vi "hipotTest.vi"() -> ()   [LabVIEW 2022 SP3]
uses:
  <vilib>/regexp/Match Regular Expression.xnode
panel:
  in  "?":bool
  out "HIPOT":bool
  out "HIPOT_R":string="FAIL"
  out "HIPOT BUFFER":string
  in  "start_hipot":bool
  in  "error in (no error)":errorcluster
  in  "VISA_TEST_L":refnum<visa-resource-name>="COM2"
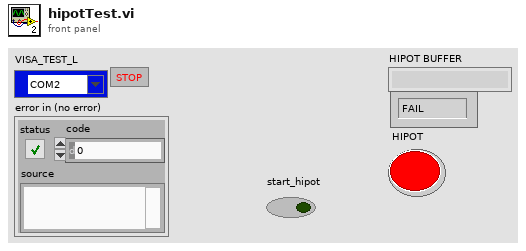
[diagram p1: front panel]
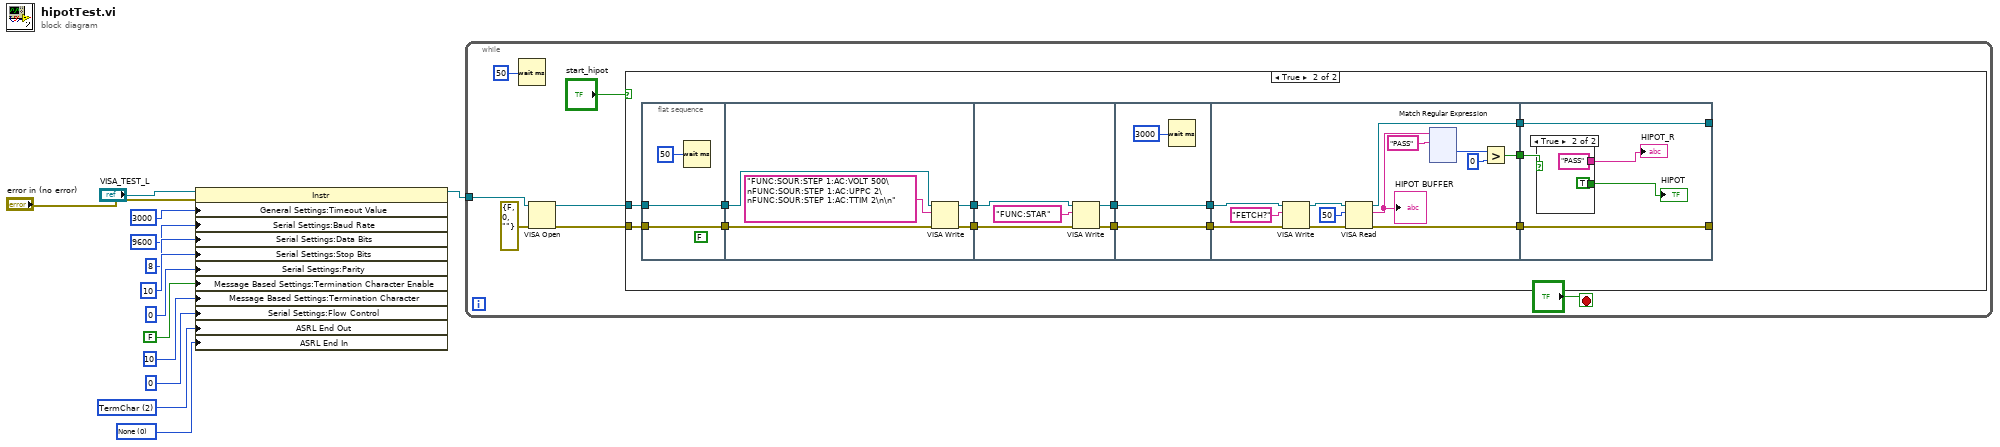
[diagram p0: block diagram]
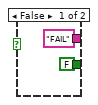
[diagram p3: hidden frame]
diagram:
  w8 = u16 0 items=["None", "Last Bit", "TermChar"] ("Serial Settings:End Mode for Reads")
  w10 = u16 2 items=["None", "Last Bit", "TermChar", "Break"] ("Serial Settings:End Mode for Writes")
  n1 = property class="Instr"(reference="VISA_TEST_L", error in="error in (no error)", "General Settings:Timeout Value"=u32 3000, "Serial Settings:Baud Rate"=u32 9600, "Serial Settings:Data Bits"=u16 8, "Serial Settings:Stop Bits"=u16 10, "Serial Settings:Parity"=u16 0, "Message Based Settings:Termination Character Enable"=FALSE ("TermChar En"), "Message Based Settings:Termination Character"=u8 10, "Serial Settings:Flow Control"=u16 0, "ASRL End Out"=w10, "ASRL End In"=w8) -> (reference out=w2:refnum<visa-resource-name>)  [unwired: 1 out]
  n2 = while {
    tunnel: w2 -> [w17]
    stop <- "?" stop-if-true
    n3 = Wait (ms)(milliseconds to wait=u32 50) -> ()  [unwired: 1 out]
    n4 = VISA Open ("VISA打开")(error in (no error)=errorcluster {"status"=FALSE, "code"=0, "source"=""}, VISA resource name=w17) -> (VISA resource name=w15:refnum<visa-resource-name>, error out=w18:errorcluster)  [unwired: 3 in]
    n5 = case shown="True" "start_hipot" {
      tunnel: w18 -> [_ w31]
      tunnel: w15 -> [_ w33]
      frame False {
      }
      frame True {
        n6 = flat-sequence {
          tunnel: w33 -> [w35]
          tunnel: [w35] -> w32
          tunnel: w31 -> [w34]
          tunnel: [w34] -> w30
          tunnel: w32 -> [w40]
          tunnel: w30 -> [w39]
          tunnel: [w38] -> w29
          tunnel: [w37] -> w28
          tunnel: w29 -> [w45]
          tunnel: w28 -> [w44]
          tunnel: [w43] -> w27
          tunnel: [w42] -> w26
          tunnel: w27 -> [w48]
          tunnel: w26 -> [w47]
          tunnel: [w48] -> w25
          tunnel: [w47] -> w24
          tunnel: w25 -> [w54]
          tunnel: w24 -> [w53]
          tunnel: [w52] -> w23
          tunnel: [w51] -> w22
          tunnel: [w50] -> w21
          tunnel: w23 -> [w184]
          tunnel: w22 -> [w183]
          tunnel: w21 -> [w180]
          tunnel: [w184] -> _
          tunnel: [w183] -> _
          frame #0 {
            (unwired) FALSE ("RST(ok)")
            n7 = Wait (ms)(milliseconds to wait=u32 50) -> ()  [unwired: 1 out]
          }
          frame #1 {
            n8 = VISA Write(VISA resource name=w40, write buffer="FUNC:SOUR:STEP 1:AC:VOLT 500\nFUNC:SOUR:STEP 1:AC:UPPC 2\nFUNC:SOUR:STEP 1:AC:TTIM 2\n\n", error in (no error)=w39) -> (VISA resource name out=w38:refnum<visa-resource-name>, error out=w37:errorcluster)  [unwired: 1 out]
          }
          frame #2 {
            n9 = VISA Write(VISA resource name=w45, write buffer="FUNC:STAR", error in (no error)=w44) -> (VISA resource name out=w43:refnum<visa-resource-name>, error out=w42:errorcluster)  [unwired: 1 out]
          }
          frame #3 {
            n10 = Wait (ms)(milliseconds to wait=u32 3000) -> ()  [unwired: 1 out]
          }
          frame #4 {
            n11 = VISA Write(VISA resource name=w54, write buffer="FETCH?", error in (no error)=w53) -> (VISA resource name out=w55:refnum<visa-resource-name>, error out=w56:errorcluster)  [unwired: 1 out]
            n12 = VISA Read(VISA resource name=w55, byte count=u32 50, error in (no error)=w56) -> (VISA resource name out=w51:refnum<visa-resource-name>, read buffer=w58:string, error out=w52:errorcluster)  [unwired: 1 out]
            "HIPOT BUFFER" <- w58
            n13 = xnode "Match Regular Expression"("input string"=w58, "regular expression"="PASS") -> ("offset past match"=w59:i32)  [unwired: 4 in, 4 out]
            n14 = Greater?(x=w59, y=0) -> (0:w50:bool)
          }
          frame #5 {
            n15 = case shown="True" w180 {
              tunnel: ["FAIL" "PASS"] -> w182
              tunnel: [FALSE TRUE] -> w181
              frame False {
              }
              frame True {
              }
            }
            "HIPOT_R" <- w182
            "HIPOT" <- w181
          }
        }
      }
    }
  }
